vi "_GetDataTypeDescription.vi"(8 "error in (no error)":errorcluster, 11 "Type Descriptor":i16[](array[numeric])) -> (0 "error out":errorcluster, 3 "String":string)   [LabVIEW 2019]
doc: "NEVSTOP-Programming-Palette 2022.3.9.1\nNEVSTOP - NEVSTOP\nCopyright (c) 2022, NEVSTOP"
uses:
  <userlib>/_OpenG.lib/lvdata/lvdata.llb/Waveform Subtype Enum__ogtk.ctl
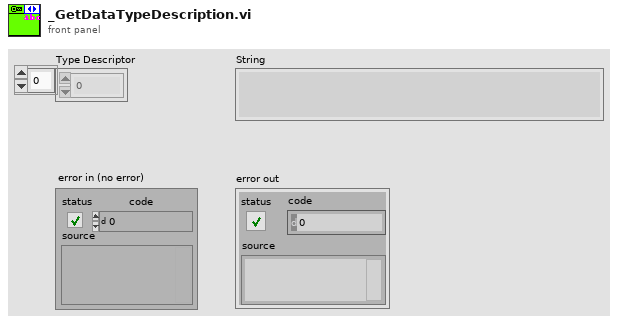
[diagram p1: front panel]
types:
  T1 = typedef "Type Descriptor Enumeration__ogtk.ctl" = enum8{"<Null>", "I8", "I16", "I32", "I64", "U8", "U16", "U32", "U64", "SGL", "DBL", "EXT", "CSG", "CDB", "CXT", "0x0F", "0x10", "0x11", "0x12", "0x13", "0x14", "Enum U8", "Enum U16", "Enum U32", "Enum U64", "SGL PQ", "DBL PQ", "EXT PQ", "CSG PQ", "CDB PQ", "CXT PQ", "0x1F", "0x20", "Boolean", "0x22", "0x23", "0x24", "0x25", "0x26", "0x27", "0x28", "0x29", "0x2A", "0x2B", "0x2C", "0x2D", "0x2E", "0x2F", "String", "0x31", "Path", "Pict", "0x34", "0x35", "0x36", "DAQ", "0x38", "0x39", "0x3A", "0x3B", "0x3C", "0x3D", "0x3E", "0x3F", "Array", "0x41", "0x42", "0x43", "0x44", "0x45", "0x46", "0x47", "0x48", "0x49", "0x4A", "0x4B", "0x4C", "0x4D", "0x4E", "0x4F", "Cluster", "0x51", "0x52", "Variant", "Waveform", "0x55", "0x56", "0x57", "0x58", "0x59", "0x5A", "0x5B", "0x5C", "0x5D", "0x5E", "Fixed Point", "0x60", "0x61", "0x62", "0x63", "0x64", "0x65", "0x66", "0x67", "0x68", "0x69", "0x6A", "0x6B", "0x6C", "0x6D", "0x6E", "0x6F", "Refnum", "0x71", "0x72", "Set Collection", "Map Collection"}
  T2 = typedef "Type Descriptor__ogtk.ctl" = i16[]
  T3 = typedef "Waveform Subtype Enum__ogtk.ctl" = enum8{"<Not a Waveform Type>", "0x01", "Analog 16-bit signed", "Analog Double-Precision", "0x04", "Analog Single Precision", "Timestamp", "Digital Data", "Digital Waveform", "Dynamic Data", "Analog Extended-Precision", "Analog 8-bit unsigned", "Analog 16-bit unsigned", "Analog 32-bit unsigned", "Analog 8-bit signed", "Analog 32-bit signed", "Analog Complex Single-Precision", "Analog Complex Double-Precision", "Analog Complex Extended Precision", "Analog 64-bit signed", "Analog 64-bit unsigned"}
  T4 = typedef "Refnum Subtype Enum__ogtk.ctl" = enum8{"Generic", "Datalog File Refnum", "Byte Stream File Refnum", "Device Refnum", "Occurence Refnum", "TCP Connection Refnum", "VISA Refnum (Obsolete)", "Automation Renum", "VI Server Refnum", "Menu Refnum", "IVI Refnum (Obsolete)", "IMAQ Session", "0x0C", "Datasocket Refnum", "VISA Resource", "IVI Logical Name", "UDP Connection Refnum", "Notifier Refnum", "Queue Refnum", "IrDA Refnum", "Hardware Plugin Refnum", "Hardware Plugin Tag Refnum", "DAQmx Refnum", "Event Registration Refnum", ".NET Refnum", "User Event Refnum", "0x1A", "Event Callback", "0x1C", "0x1D", "LabVIEW Class Instance", "Bluetooth", "Data Value References", "RT FIFO", "TDM Streaming"}
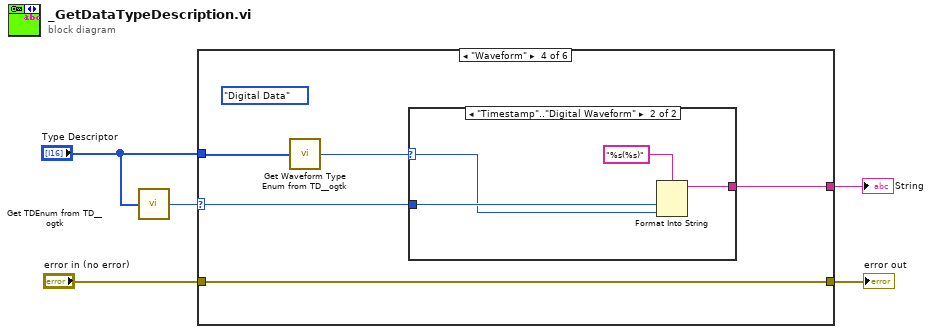
[diagram p0: block diagram]
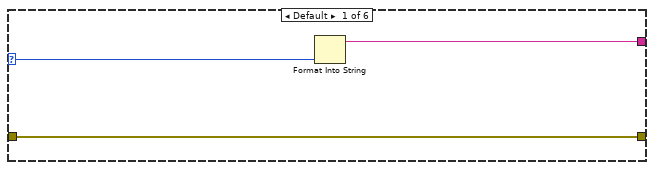
[diagram p2: hidden frame]
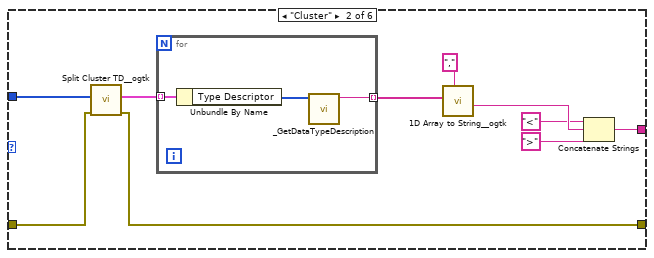
[diagram p3: hidden frame]
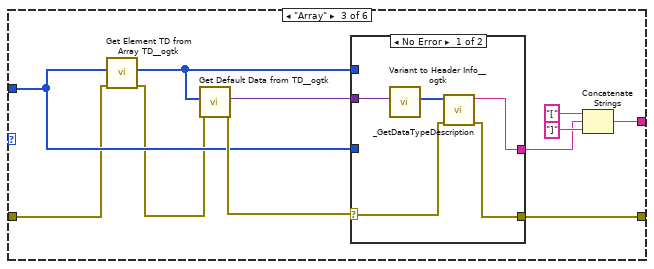
[diagram p4: hidden frame]
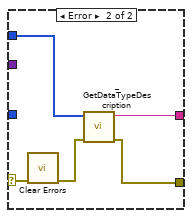
[diagram p5: hidden frame]
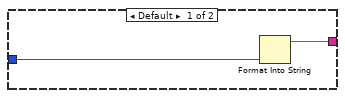
[diagram p6: hidden frame]
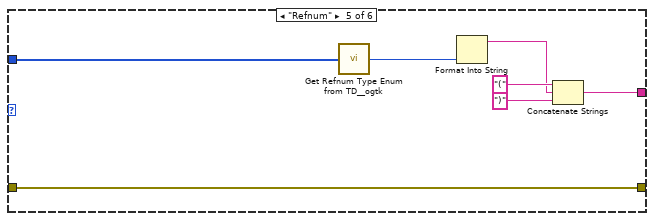
[diagram p7: hidden frame]
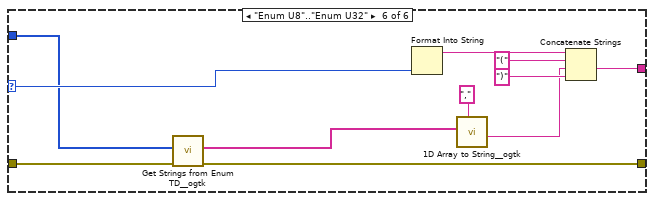
[diagram p8: hidden frame]
diagram:
  n1 = call <userlib>:"Get TDEnum from TD__ogtk.vi"("Type Descriptor"="Type Descriptor") -> ("Type Descriptor Enumeration"=w5:T1)  [unwired: 4 in]
  n2 = case shown="\"Waveform\"" w5 {
    selector: w5 -> [w8 _ _ w44 _ w68]
    tunnel: "Type Descriptor" -> [_ w12 w26 w46 w55 w64]
    tunnel: [w7 w15 w32 w43 w57 w69] -> w4
    tunnel: [w6 w9 w22 w47 w54 w61] -> w2
    tunnel: "error in (no error)" -> [w6 w10 w24 w47 w54 w62]
    frame Default {
      n3 = Format Into String(w8) -> (resulting string=w7:string)  [unwired: 3 in, 1 out]
    }
    frame "Cluster" {
      n4 = call <userlib>:"Split Cluster TD__ogtk.vi"("error in (no error)"=w10, "Type Descriptor"=w12) -> ("error out"=w9:errorcluster, "Type Descriptors"=w11:cluster{"Type Descriptor":T2}[])  [unwired: 8 in]
      n5 = for {
        tunnel: [w20] -> w18 mode=indexing
        tunnel: w11 -> [w21] mode=indexing
        n6 = Unbundle By Name(w21) -> ("Type Descriptor"=w19:T2)
        n7 = call "_GetDataTypeDescription.vi"("Type Descriptor"=w19) -> ("String"=w20:string)  [unwired: 9 in, 1 out]
      }
      n8 = call <userlib>:"1D Array to String__ogtk.vi"("delimiter (Tab)"=",", "Array of Strings"=w18) -> ("delimited string"=w16:string)  [unwired: 9 in]
      n9 = Concatenate Strings("<" ("string"), w16, ">" ("string")) -> (w15:string)
    }
    frame "Array" {
      n10 = call <userlib>:"Get Element TD from Array TD__ogtk.vi"("error in (no error)"=w24, "Array Type Descriptor"=w26) -> ("error out"=w23:errorcluster, "Element Type Descriptor"=w25:T2)  [unwired: 8 in]
      n11 = call <userlib>:"Get Default Data from TD__ogtk.vi"("error in (no error)"=w23, "Type Descriptor"=w25) -> ("error out"=w27:errorcluster, "Default VData"=w28:variant)  [unwired: 8 in]
      n12 = case shown="No Error" w27 {
        selector: w27 -> [w34 w39]
        tunnel: [w37 w42] -> w29
        tunnel: w28 -> [w36 _]
        tunnel: w26 -> [_ _]
        tunnel: w25 -> [_ w41]
        tunnel: [w33 w40] -> w22
        frame No Error {
          n13 = call <userlib>:"Variant to Header Info__ogtk.vi"("Variant"=w36) -> ("Type Descriptor"=w35:T2)  [unwired: 3 in, 2 out]
          n14 = call "_GetDataTypeDescription.vi"("error in (no error)"=w34, "Type Descriptor"=w35) -> ("error out"=w33:errorcluster, "String"=w37:string)  [unwired: 8 in]
        }
        frame Error {
          n15 = call <vilib>:"Clear Errors.vi"("error in (no error)"=w39) -> ("error out"=w38:errorcluster)  [unwired: 5 in, 1 out]
          n16 = call "_GetDataTypeDescription.vi"("error in (no error)"=w38, "Type Descriptor"=w41) -> ("error out"=w40:errorcluster, "String"=w42:string)  [unwired: 8 in]
        }
      }
      n17 = Concatenate Strings("[" ("string"), w29, "]" ("string")) -> (w32:string)
    }
    frame "Waveform" {
      (unwired) Waveform_Subtype_Enum__ogtk."Digital Data" ("Waveform Subtype Enum")
      n18 = call <userlib>:"Get Waveform Type Enum from TD__ogtk.vi"("Type Descriptor"=w46) -> ("Waveform Subtype Enum"=w45:T3)  [unwired: 4 in]
      n19 = case shown="\"Timestamp\"..\"Digital Waveform\"" w45 {
        selector: w45 -> [_ w50]
        tunnel: w44 -> [w48 w51]
        tunnel: [w49 w53] -> w43
        frame Default {
          n20 = Format Into String(w48) -> (resulting string=w49:string)  [unwired: 3 in, 1 out]
        }
        frame "Timestamp".."Digital Waveform" {
          n21 = Format Into String(format string="%s(%s)", w51, w50) -> (resulting string=w53:string)  [unwired: 2 in, 1 out]
        }
      }
    }
    frame "Refnum" {
      n22 = call <userlib>:"Get Refnum Type Enum from TD__ogtk.vi"("Type Descriptor"=w55) -> ("Refnum Subtype Enum"=w56:T4)  [unwired: 4 in]
      n23 = Format Into String(w56) -> (resulting string=w58:string)  [unwired: 3 in, 1 out]
      n24 = Concatenate Strings("(" ("string"), w58, ")" ("string")) -> (w57:string)
    }
    frame "Enum U8".."Enum U32" {
      n25 = call <userlib>:"Get Strings from Enum TD__ogtk.vi"("error in (no error)"=w62, "Type Descriptor"=w64) -> ("error out"=w61:errorcluster, "enum strings"=w63:string[])  [unwired: 7 in, 1 out]
      n26 = Format Into String(w68) -> (resulting string=w67:string)  [unwired: 3 in, 1 out]
      n27 = call <userlib>:"1D Array to String__ogtk.vi"("delimiter (Tab)"=",", "Array of Strings"=w63) -> ("delimited string"=w65:string)  [unwired: 9 in]
      n28 = Concatenate Strings(w67, "(" ("string"), w65, ")" ("string")) -> (w69:string)
    }
  }
  "String" <- w4
  "error out" <- w2
